vi "Deploy to Platform.vi"(8 "error in (no error)":errorcluster, 9 "Processed VIA":string, 10 "Platform":string, 11 "TargetPluginManager in":refnum<class "PlatformPluginManager.lvclass">) -> (0 "error out":errorcluster, 1 "Processed VIA":string, 2 "Deployed Resource":string, 3 "TargetPluginManager out":refnum<class "PlatformPluginManager.lvclass">, 5 "Response":string)   [LabVIEW 2020, in "PicoG-Core.lvlib" / "PlatformPluginManager.lvclass"]
uses:
  PlatformPluginManager.lvclass
  DeployPlatform/DeployPlatform.lvclass
  DeployResource/DeployResource.lvclass
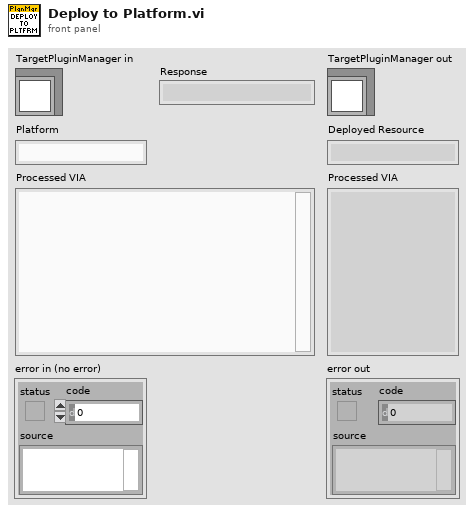
[diagram p1: front panel]
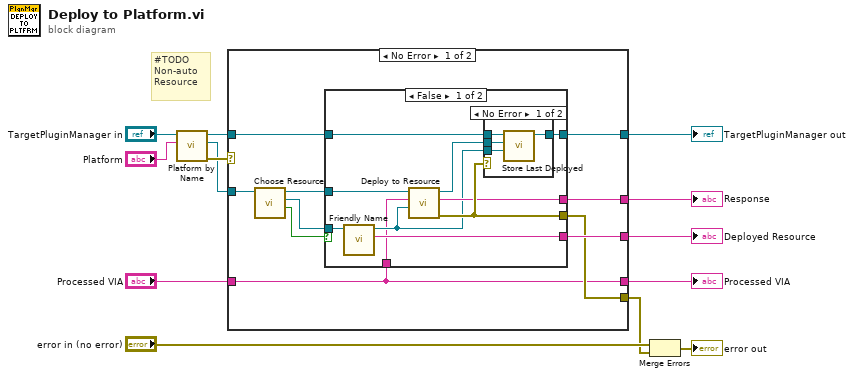
[diagram p0: block diagram]
diagram:
  # "#TODO\nNon-auto Resource"
  n1 = call "Platform by Name.vi"("Platform"="Platform", "TargetPluginManager in"="TargetPluginManager in") -> ("error out"=w9:errorcluster, "Target"=w1:refnum<class "DeployPlatform.lvclass">, "TargetPluginManager out"=w10:refnum<class "PlatformPluginManager.lvclass">)  [unwired: 7 in]
  n2 = case shown="No Error" w9 {
    selector: w9 -> [_ w41]
    tunnel: w10 -> [w18 w40]
    tunnel: w1 -> [w23 _]
    tunnel: "Processed VIA" -> [w17 _]
    tunnel: [w20 w41] -> w6
    tunnel: [w22 w40] -> w5
    tunnel: [w17 _] -> w4
    tunnel: [w21 _] -> w3
    tunnel: [w19 _] -> w2
    frame No Error {
      n3 = call-dynamic "Choose Resource.vi"("DeployTarget in"=w23) -> ("Cancelled"=w15:bool, "Resource"=w16:refnum<class "DeployResource.lvclass">, "DeployTarget out"=w14:refnum<class "DeployPlatform.lvclass">)  [unwired: 7 in, 1 out]
      n4 = case shown="False" w15 {
        tunnel: w16 -> [w32 _]
        tunnel: w18 -> [w29 w39]
        tunnel: [w28 w39] -> w22
        tunnel: [w31 _] -> w21
        tunnel: w14 -> [w27 _]
        tunnel: w17 -> [w24 _]
        tunnel: [w33 _] -> w20
        tunnel: [w30 _] -> w19
        frame False {
          n5 = call-dynamic "Friendly Name.vi"("DeployResource in"=w32) -> ("Friendly Name"=w31:string, "DeployResource out"=w25:refnum<class "DeployResource.lvclass">)  [unwired: 8 in, 1 out]
          n6 = call-dynamic "Deploy to Resource.vi"("Resource"=w25, "VIA"=w24, "DeployTarget in"=w27) -> ("error out"=w33:errorcluster, "Response"=w30:string, "DeployTarget out"=w26:refnum<class "DeployPlatform.lvclass">)  [unwired: 6 in]
          n7 = case shown="No Error" w33 {
            tunnel: w29 -> [w37 w38]
            tunnel: [w36 w38] -> w28
            tunnel: w25 -> [w35 _]
            tunnel: w26 -> [w34 _]
            frame No Error {
              n8 = call "Store Last Deployed.vi"("PicoG-Core:DeployResource"=w35, "PicoG-Core:DeployTarget"=w34, "TargetPluginManager in"=w37) -> ("TargetPluginManager out"=w36:refnum<class "PlatformPluginManager.lvclass">)  [unwired: 7 in, 1 out]
            }
            frame Error {
            }
          }
        }
        frame True {
        }
      }
    }
    frame Error {
    }
  }
  "TargetPluginManager out" <- w5
  "Processed VIA" <- w4
  "Deployed Resource" <- w3
  "Response" <- w2
  n9 = Merge Errors("error in (no error)", w6) -> (→"error out":errorcluster)
